vi "isProtocolName.vi"(8 "error in (no error)":errorcluster, 10 "name":string, 11 "Protocol_Generic in":refnum<class "Protocol_Generic.lvclass">) -> (0 "error out":errorcluster, 2 "isName":bool, 3 "Protocol_Generic out":refnum<class "Protocol_Generic.lvclass">)   [LabVIEW 2015, in "Protocol_Generic.lvclass"]
uses:
  Protocol_Generic.lvclass
  Protocol_Generic.lvclass/Protocol_Generic.ctl
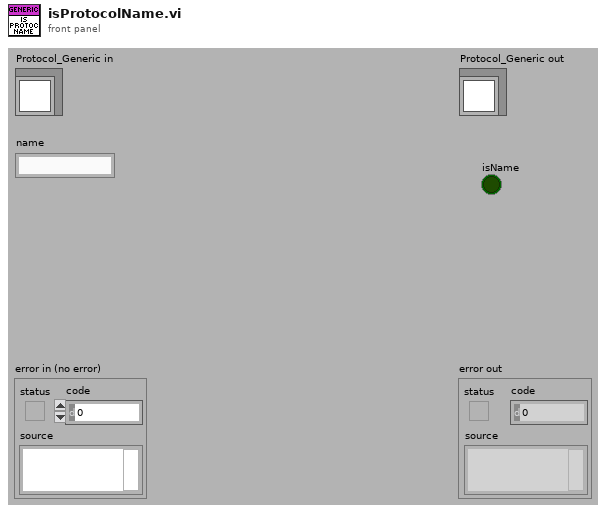
[diagram p1: front panel]
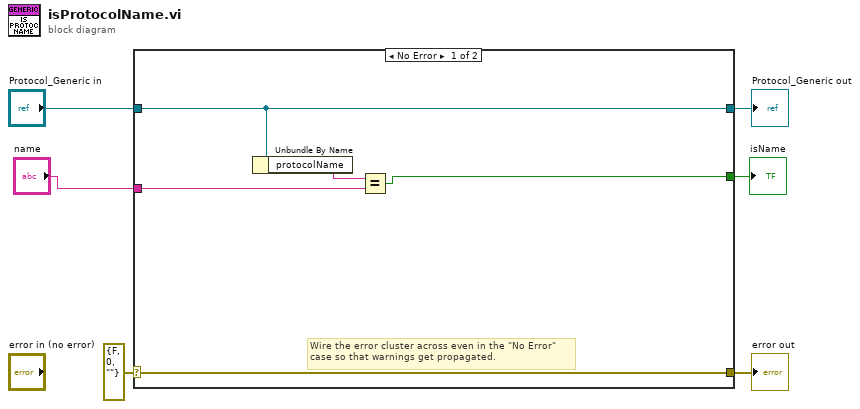
[diagram p0: block diagram]
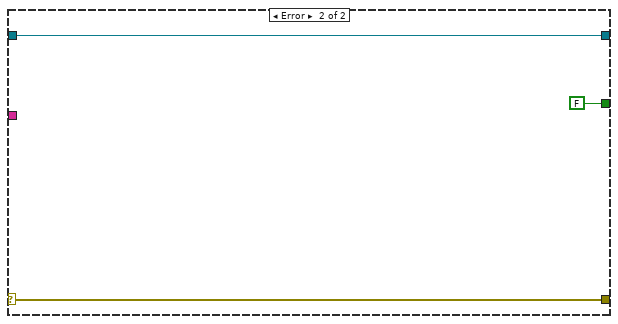
[diagram p2: hidden frame]
diagram:
  n1 = case shown="No Error" errorcluster {"status"=FALSE, "code"=0, "source"=""} ("error IO") {
    selector: errorcluster {"status"=FALSE, "code"=0, "source"=""} ("error IO") -> [w11 w14]
    tunnel: [w11 w14] -> w6
    tunnel: [w10 w13] -> w4
    tunnel: "Protocol_Generic in" -> [w10 w13]
    tunnel: "name" -> [w8 _]
    tunnel: [w7 FALSE] -> w2
    frame No Error {
      # "Wire the error cluster across even in the \"No Error\"\ncase so that warnings get propagated."
      n2 = Unbundle By Name(w10) -> ("protocolName"=w9:string)
      n3 = Equal?(x=w9, y=w8) -> (x = y?=w7:bool)
    }
    frame Error {
    }
  }
  "error out" <- w6
  "Protocol_Generic out" <- w4
  "isName" <- w2
